vi "SmartSEM Remote API get SEM HV data.vi"(8 "error in":errorcluster, 11 "ActiveX Container":refnum<k7>(container)) -> (0 "error out":errorcluster, 2 "SEM HV Data Output":T1 {"Sys Vac (Torr)" format="%.2e"; "Gun Vac (Torr)" format="%.2e"; "Supp Monitor (V)" format="%.1f"; "Liner Actual (V)" format="%.1f"; "Fil I Actual (A)" format="%.3f"; "Ext Actual (V)" format="%.1f"; "Supp Actual (V)" format="%.1f"; "EHT Actual (V)" format="%.1f"; "EHT Target (V)" format="%.1f"; "Liner Target (V)" format="%.1f"; "Fil I Target (A)" format="%.3f"; "Fil Age (hr)" format="%.2f"; "Ext I Actual (uA)" format="%.1f"; "Ext Target (V)" format="%.1f"}, 3 "reference out":refnum<k7>)   [LabVIEW 2018]
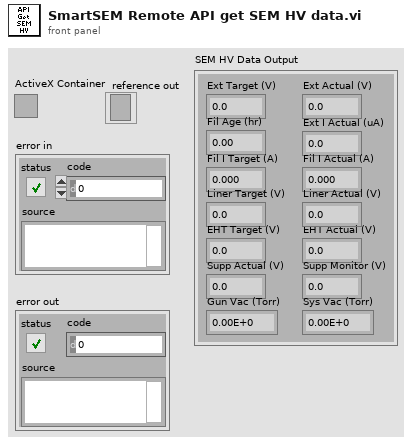
[diagram p1: front panel]
types:
  T1 = cluster{"Ext Target (V)":sgl, "Ext Actual (V)":sgl, "Fil Age (hr)":sgl, "Ext I Actual (uA)":sgl, "Fil I Target (A)":sgl, "Fil I Actual (A)":sgl, "Liner Target (V)":sgl, "Liner Actual (V)":sgl, "EHT Target (V)":sgl, "EHT Actual (V)":sgl, "Supp Actual (V)":sgl, "Supp Monitor (V)":sgl, "Gun Vac (Torr)":sgl, "Sys Vac (Torr)":sgl}
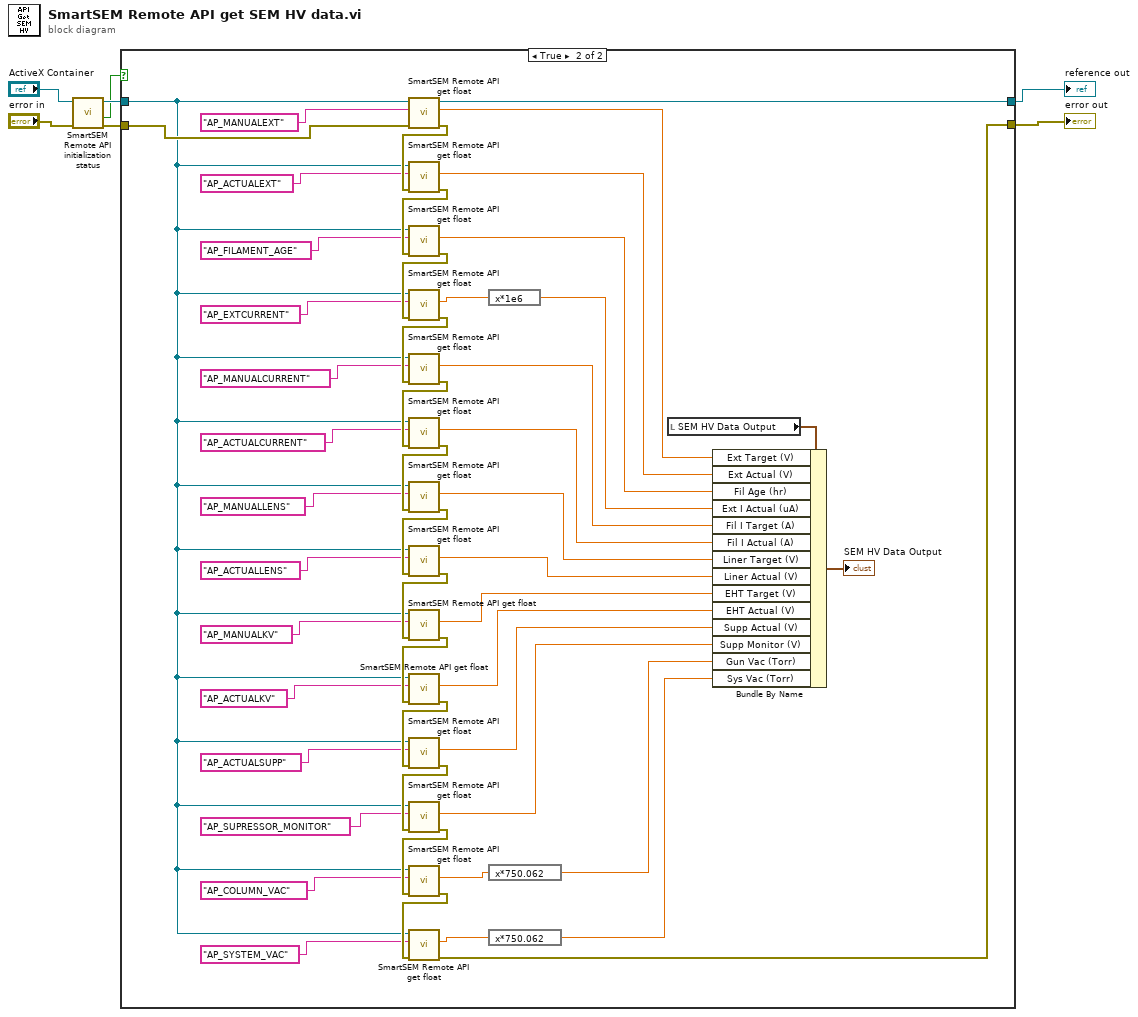
[diagram p0: block diagram]
diagram:
  n1 = call "SmartSEM Remote API initialization status.vi"("error in"="error in", "ActiveX Container"="ActiveX Container") -> ("error out"=w4:errorcluster, "API initialized"=w3:bool, "reference out"=w5:refnum<k7>)  [unwired: 7 in]
  n2 = case shown="True" w3 {
    tunnel: w5 -> [w9 w10]
    tunnel: w4 -> [w8 w41]
    tunnel: [w9 w12] -> w7
    tunnel: [w8 w11] -> w6
    frame False {
    }
    frame True {
      n3 = call "SmartSEM Remote API get float.vi"("error in"=w41, "lpszParam"="AP_MANUALEXT", "ActiveX Container"=w10) -> ("error out"=w42:errorcluster, "vValue"=w23:sgl, "reference out"=w12:refnum<k7>)  [unwired: 6 in]
      n4 = call "SmartSEM Remote API get float.vi"("error in"=w42, "lpszParam"="AP_ACTUALEXT", "ActiveX Container"=w10) -> ("error out"=w43:errorcluster, "vValue"=w22:sgl)  [unwired: 6 in, 1 out]
      n5 = call "SmartSEM Remote API get float.vi"("error in"=w43, "lpszParam"="AP_FILAMENT_AGE", "ActiveX Container"=w10) -> ("error out"=w44:errorcluster, "vValue"=w21:sgl)  [unwired: 6 in, 1 out]
      n6 = call "SmartSEM Remote API get float.vi"("error in"=w44, "lpszParam"="AP_EXTCURRENT", "ActiveX Container"=w10) -> ("error out"=w45:errorcluster, "vValue"=w24:sgl)  [unwired: 6 in, 1 out]
      n7 = call "SmartSEM Remote API get float.vi"("error in"=w45, "lpszParam"="AP_MANUALCURRENT", "ActiveX Container"=w10) -> ("error out"=w46:errorcluster, "vValue"=w20:sgl)  [unwired: 6 in, 1 out]
      n8 = call "SmartSEM Remote API get float.vi"("error in"=w46, "lpszParam"="AP_ACTUALCURRENT", "ActiveX Container"=w10) -> ("error out"=w52:errorcluster, "vValue"=w19:sgl)  [unwired: 6 in, 1 out]
      n9 = call "SmartSEM Remote API get float.vi"("error in"=w52, "lpszParam"="AP_MANUALLENS", "ActiveX Container"=w10) -> ("error out"=w51:errorcluster, "vValue"=w18:sgl)  [unwired: 6 in, 1 out]
      n10 = call "SmartSEM Remote API get float.vi"("error in"=w51, "lpszParam"="AP_ACTUALLENS", "ActiveX Container"=w10) -> ("error out"=w50:errorcluster, "vValue"=w17:sgl)  [unwired: 6 in, 1 out]
      n11 = call "SmartSEM Remote API get float.vi"("error in"=w50, "lpszParam"="AP_MANUALKV", "ActiveX Container"=w10) -> ("error out"=w49:errorcluster, "vValue"=w16:sgl)  [unwired: 6 in, 1 out]
      n12 = call "SmartSEM Remote API get float.vi"("error in"=w49, "lpszParam"="AP_ACTUALKV", "ActiveX Container"=w10) -> ("error out"=w48:errorcluster, "vValue"=w15:sgl)  [unwired: 6 in, 1 out]
      n13 = call "SmartSEM Remote API get float.vi"("error in"=w48, "lpszParam"="AP_ACTUALSUPP", "ActiveX Container"=w10) -> ("error out"=w47:errorcluster, "vValue"=w14:sgl)  [unwired: 6 in, 1 out]
      n14 = call "SmartSEM Remote API get float.vi"("error in"=w47, "lpszParam"="AP_SUPRESSOR_MONITOR", "ActiveX Container"=w10) -> ("error out"=w54:errorcluster, "vValue"=w13:sgl)  [unwired: 6 in, 1 out]
      n15 = call "SmartSEM Remote API get float.vi"("error in"=w54, "lpszParam"="AP_COLUMN_VAC", "ActiveX Container"=w10) -> ("error out"=w53:errorcluster, "vValue"=w25:sgl)  [unwired: 6 in, 1 out]
      n16 = call "SmartSEM Remote API get float.vi"("error in"=w53, "lpszParam"="AP_SYSTEM_VAC", "ActiveX Container"=w10) -> ("error out"=w11:errorcluster, "vValue"=w26:sgl)  [unwired: 6 in, 1 out]
      n17 = expression code="x*1e6"(w24) -> (w55:sgl)
      n18 = expression code="x*750.062"(w25) -> (w58:sgl)
      n19 = expression code="x*750.062"(w26) -> (w57:sgl)
      n20 = local read "SEM HV Data Output"() -> (w59:T1)
      n21 = Bundle By Name(cluster=w59, "Ext Target (V)"=w23, "Ext Actual (V)"=w22, "Fil Age (hr)"=w21, "Ext I Actual (uA)"=w55, "Fil I Target (A)"=w20, "Fil I Actual (A)"=w19, "Liner Target (V)"=w18, "Liner Actual (V)"=w17, "EHT Target (V)"=w16, "EHT Actual (V)"=w15, "Supp Actual (V)"=w14, "Supp Monitor (V)"=w13, "Gun Vac (Torr)"=w58, "Sys Vac (Torr)"=w57) -> (→"SEM HV Data Output":T1)
    }
  }
  "error out" <- w6
  "reference out" <- w7
